vi "Panel.vi"(11 "NumRangeBoolEditorPanel in":refnum<class "NumRangeBoolEditorPanel.lvclass">) -> ()   [LabVIEW 2020, in "VolatusGUIControls.lvlib" / "NumRangeBoolEditorPanel.lvclass"]
uses:
  NumRangeBoolEditorPanel.lvclass
  NumRangeBoolEditorPanel.lvclass/NumRangeBoolEditorPanel.ctl
  lv-oopanel/OOPanel/Panel/Basic UI State.ctl
  lv-oopanel/OOPanel/Panel/Panel.lvclass
  lv-oopanel/OOPanel/OOPanel.lvlib
  VolatusGUIEditorCore/ElementEditorPanel/ElementEditorPanel.lvclass
  lv-autocomplete/AutoComplete/AutoComplete/AutoComplete.lvclass
  VolatusGUIEditorCore/VolatusGUIEditorCore.lvlib
  C:/dev/lv20CE/relink/volatus-gui-controls/VolatusGUIEditorCore/ElementEditorPanel/ElementEditorPanel.lvclass
  C:/dev/lv20CE/relink/lv-oopanel/OOPanel/Panel/Panel.lvclass
  C:/dev/lv20CE/relink/volatus-gui-controls/VolatusGUIControls/NumRangeBoolEditorPanel/NumRangeBoolEditorPanel.lvclass
panel:
  in  "Top":i32
  in  "Left":i32
  in  "Height":u16
  in  "Width":u16
  in  "Label Text Color":u32(colorbox) caption="Color"
  in  "Label Visible":bool caption="Visible"
  in  "Label":string
  in  "Channel":string
  in  "True Color":u32(colorbox)
  in  "False Color":u32(colorbox)
  in  "High":dbl
  in  "Low":dbl
  # "Label"
  # "Out of Range"
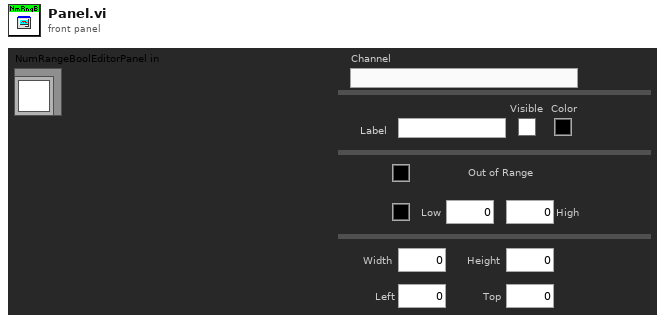
[diagram p1: front panel]
types:
  T1 = typedef "OOPanel.lvlib/Panel.lvclass/Basic UI State.ctl" = enum16{"Init", "Run", "Close"}
  T2 = typedef "VolatusGUIEditorCore.lvlib/ElementEditorPanel.lvclass/Incoming Events.ctl" = cluster{"Update Control":refnum<user-event>}
  T3 = typedef "OOPanel.lvlib/Panel.lvclass/Panel Events.ctl" = cluster{"Visbility":refnum<user-event>, "Close":refnum<user-event>}
  T4 = typedef "VolatusGUIControls.lvlib/NumRangeBoolEditorPanel.lvclass/Props.ctl" = cluster{"JSON":T5, "Label Props":T6, "Position Props":T7, "Boolean Colors Props":T8, "Width":u16, "Height":u16}
  T5 = typedef "VolatusGUIControls.lvlib/NumRangeBoolEditorPanel.lvclass/JSON Props.ctl" = cluster{"Channel":string, "Low":dbl, "High":dbl}
  T6 = typedef "VolatusGUIEditorCore.lvlib/Label Props.ctl" = cluster{"Text":string, "Text Color":u32, "Visible":bool}
  T7 = typedef "VolatusGUIEditorCore.lvlib/Position Props.ctl" = cluster{"Left":i32, "Top":i32}
  T8 = typedef "VolatusGUIEditorCore.lvlib/Boolean Color Props.ctl" = cluster{"False":u32, "True":u32}
  T9 = typedef "OOPanel.lvlib/Visibility State.ctl" = enum16{"Idle", "Closed", "Hidden", "Visible", "Subpanel", "Hidden Subpanel"}
  T10 = cluster{"Label":string, "Label Text Color":u32, "Label Visible":bool}
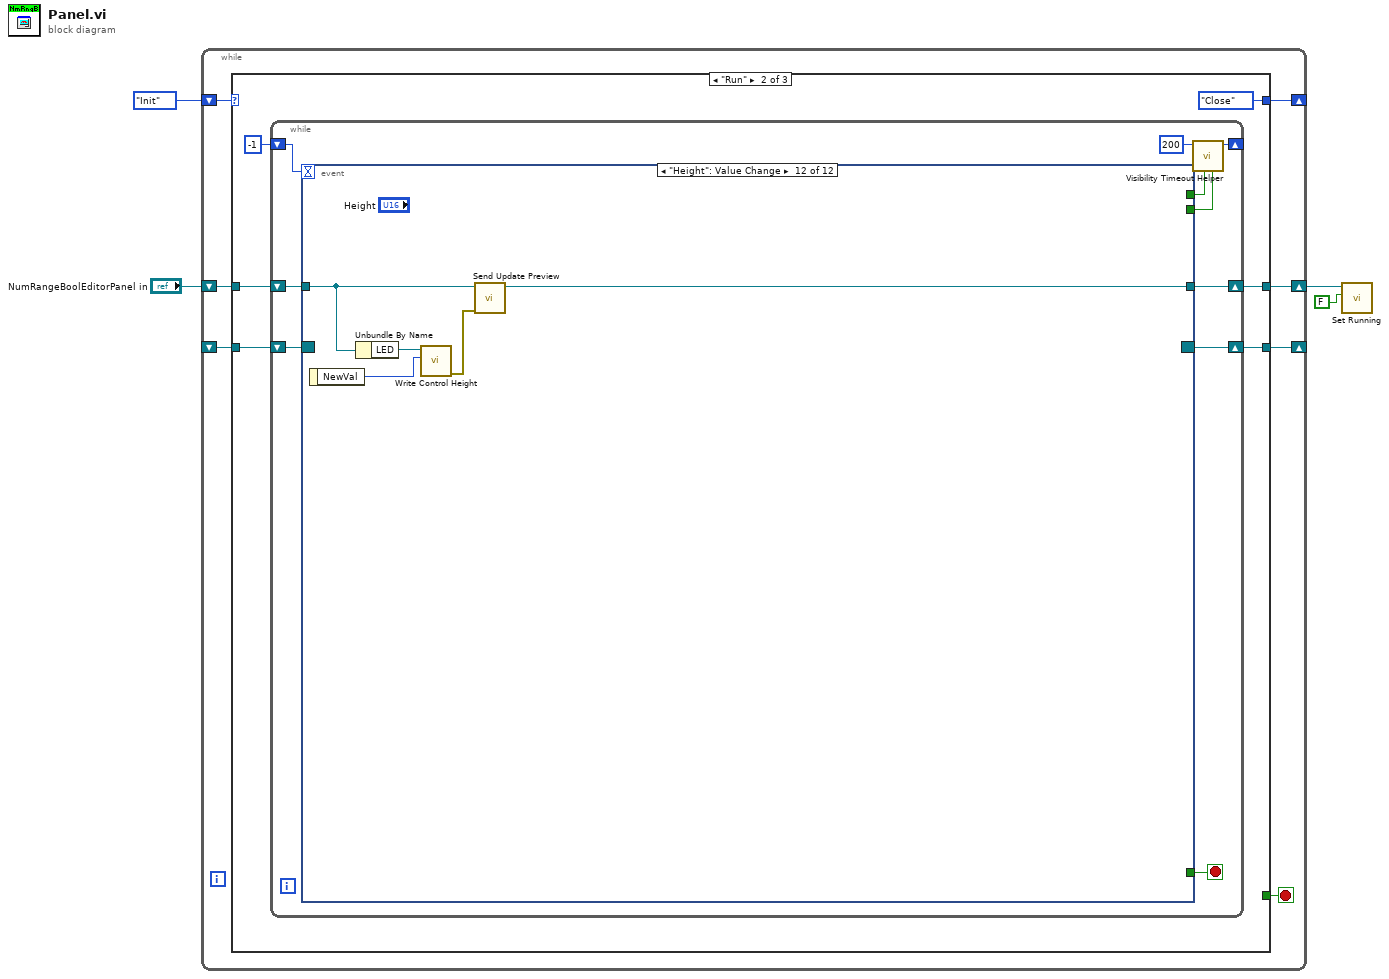
[diagram p0: block diagram]
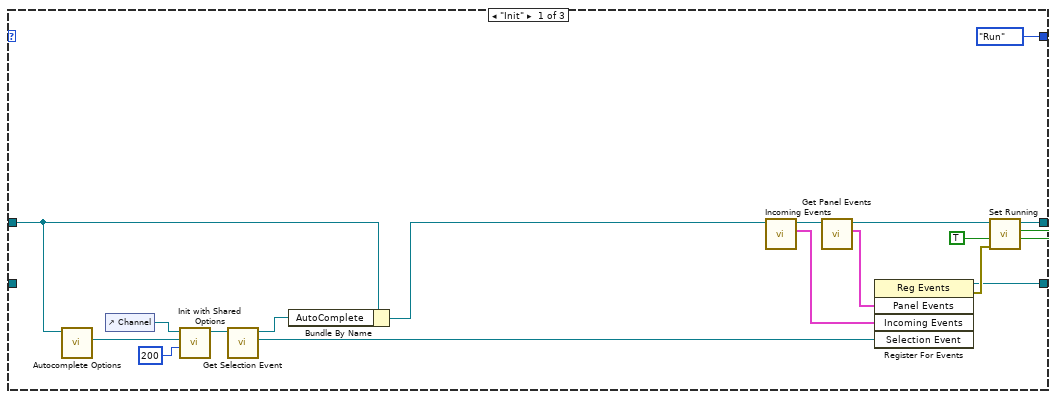
[diagram p2: hidden frame]
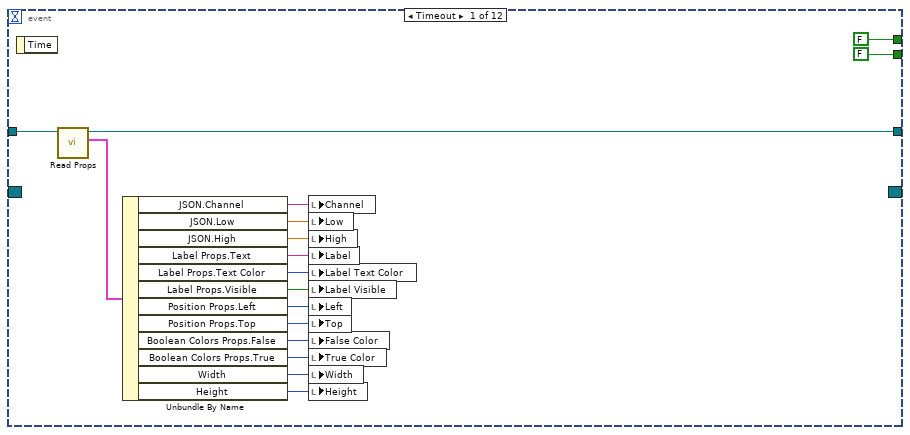
[diagram p3: hidden frame]
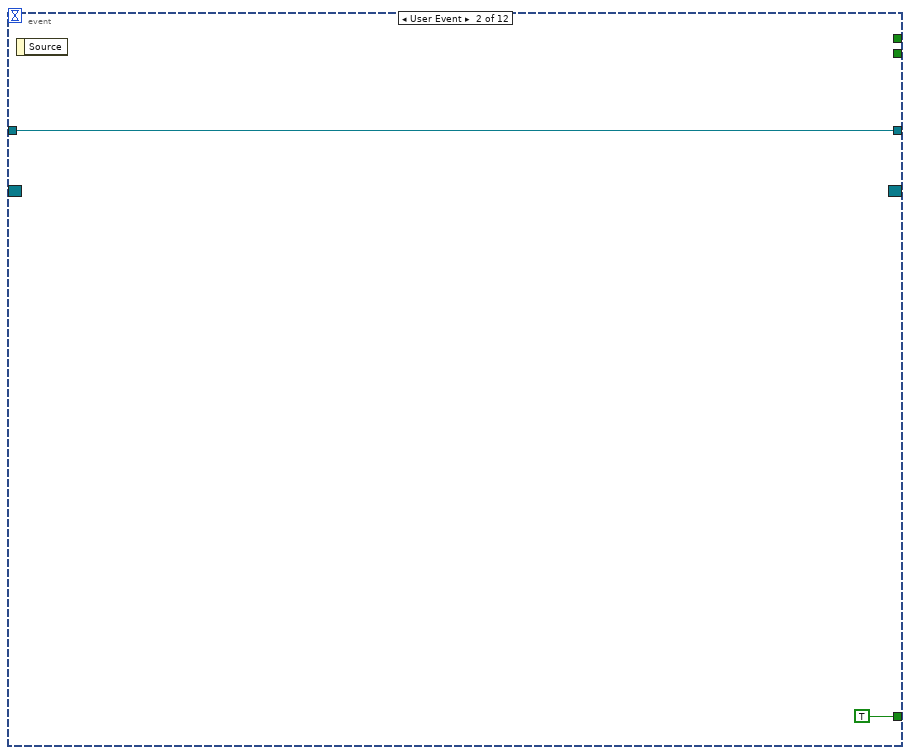
[diagram p4: hidden frame]
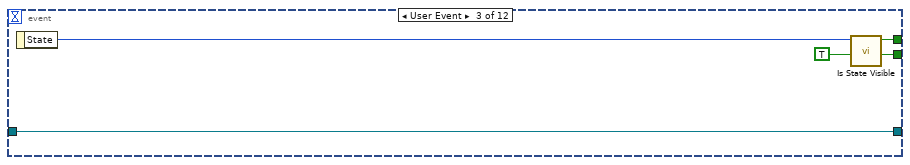
[diagram p5: hidden frame]
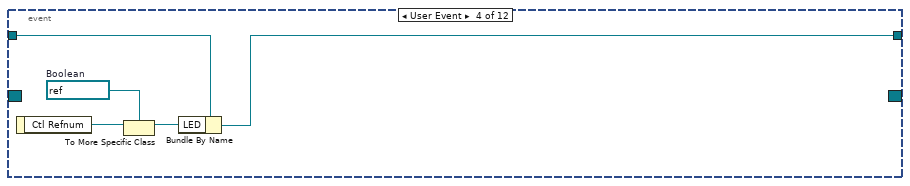
[diagram p6: hidden frame]
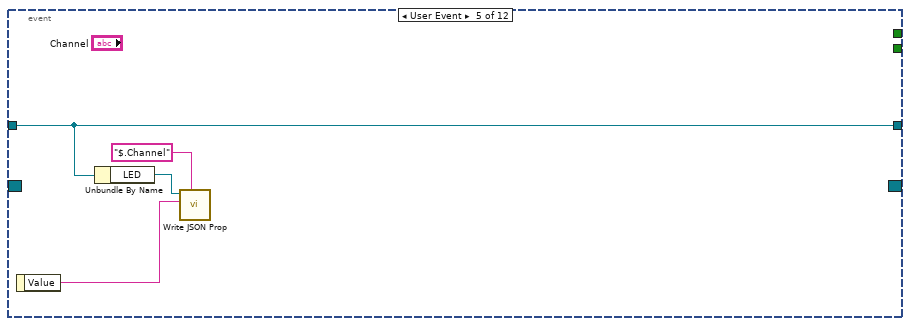
[diagram p7: hidden frame]
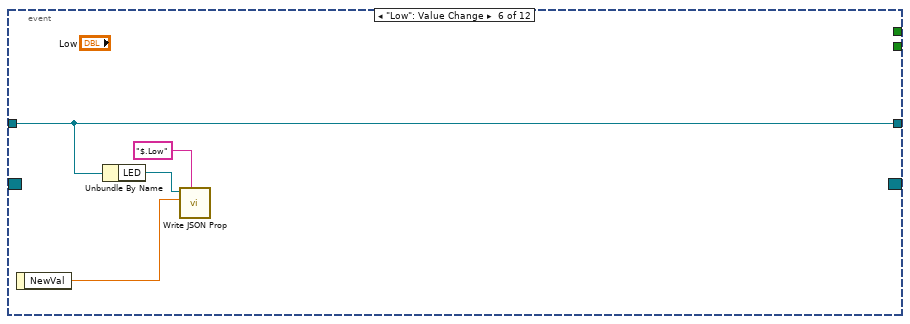
[diagram p8: hidden frame]
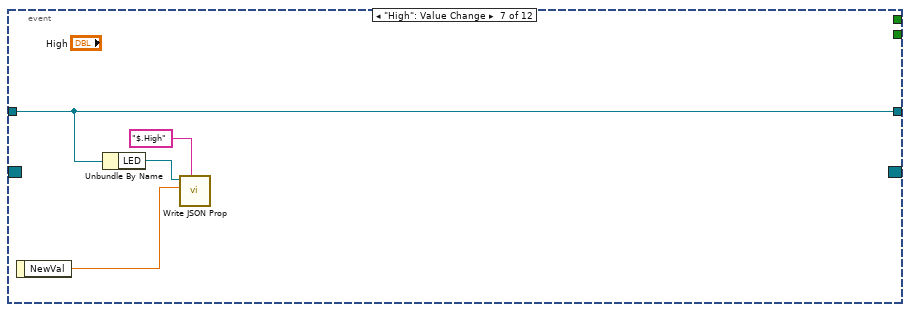
[diagram p9: hidden frame]
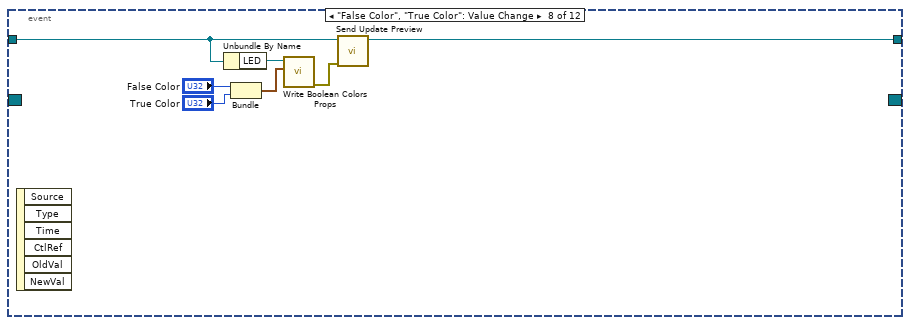
[diagram p10: hidden frame]
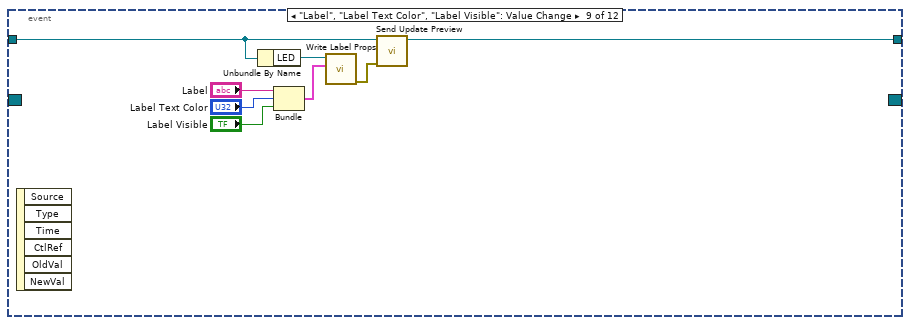
[diagram p11: hidden frame]
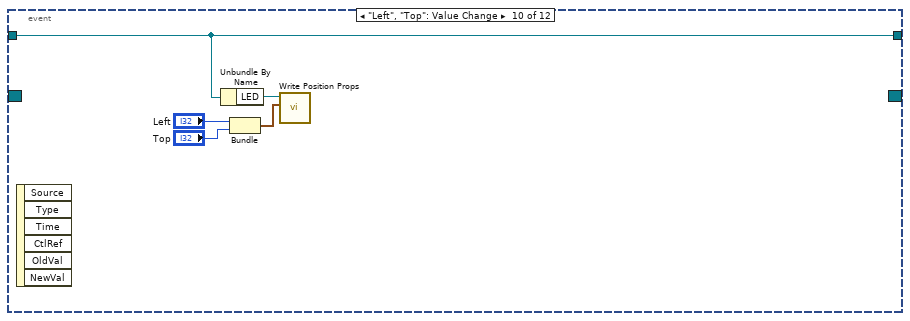
[diagram p12: hidden frame]
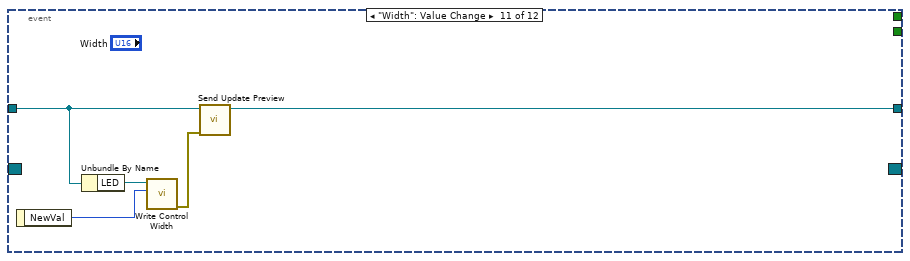
[diagram p13: hidden frame]
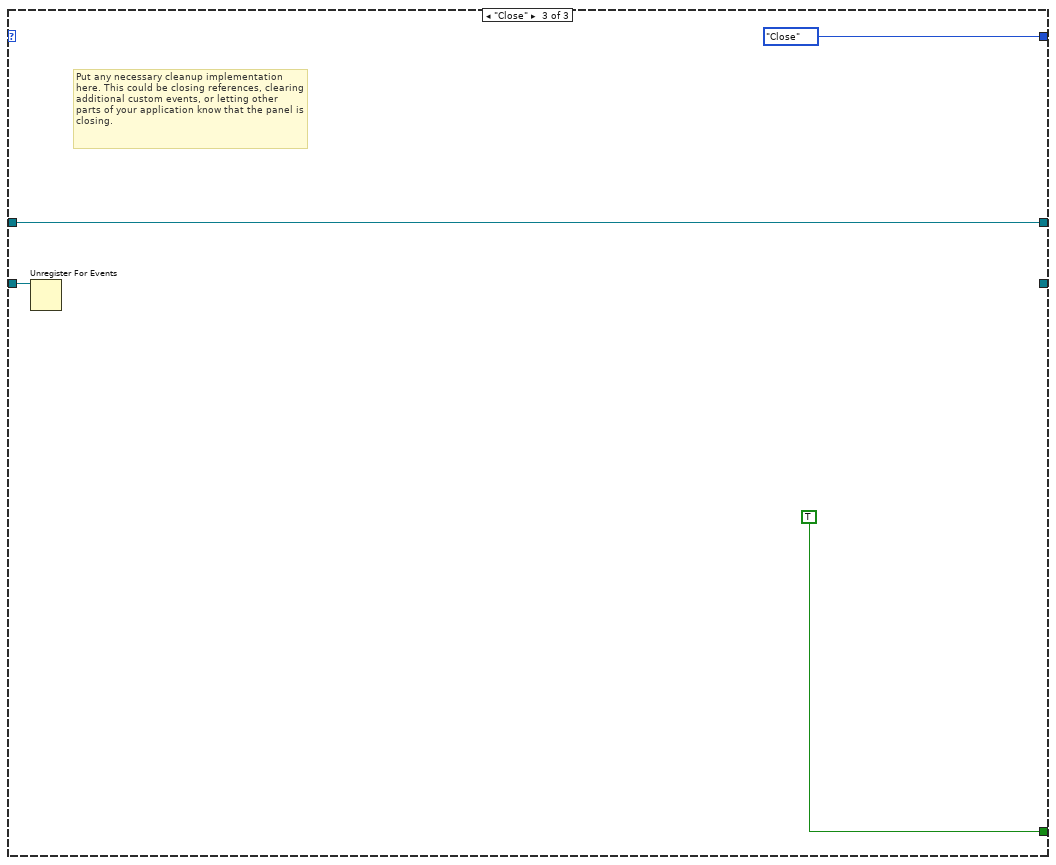
[diagram p14: hidden frame]
diagram:
  n1 = while {
    shift-right: [w10] -> _
    shift-left: _ -> [w11]
    shift-right: [w8] -> _
    shift-left: Basic_UI_State."Init" ("Basic UI State") -> [w9]
    shift-right: [w6] -> w4
    shift-left: "NumRangeBoolEditorPanel in" -> [w5]
    stop <- w7 stop-if-true
    n2 = case shown="\"Run\"" w9 {
      tunnel: w11 -> [_ w34 w116]
      tunnel: [w25 w32 _] -> w10
      tunnel: [Basic_UI_State."Run" ("Basic UI State") Basic_UI_State."Close" ("Basic UI State") Basic_UI_State."Close" ("Basic UI State")] -> w8
      tunnel: [_ _ TRUE] -> w7
      tunnel: [w24 w29 w115] -> w6
      tunnel: w5 -> [w17 w30 w115]
      frame "Init" {
        n3 = call "Autocomplete Options.vi"("ElementEditorPanel in"=w17) -> ("Autocomplete Options"=w19:refnum<class "Shared Options.lvclass">)  [unwired: 10 in]
        n4 = control-ref of="Channel"() -> (w16:refnum<vi>)
        n5 = call "Init with Shared Options.vi"("Height (200)"=i16 200, "Shared Options"=w19, "Str Refnum"=w16) -> ("AutoComplete out"=w15:refnum<class "AutoComplete.lvclass">)  [unwired: 7 in, 1 out]
        n6 = call "Get Selection Event.vi"("AutoComplete in"=w15) -> ("Selection Event"=w14:refnum<user-event>, "AutoComplete"=w12:refnum<class "AutoComplete.lvclass">)  [unwired: 9 in]
        n7 = Bundle By Name(cluster=w17, "AutoComplete"=w12) -> (w13:refnum<class "NumRangeBoolEditorPanel.lvclass">)
        n8 = call "Incoming Events.vi"("ElementEditorPanel in"=w13) -> ("Incoming Events"=w20:T2, "ElementEditorPanel out"=w21:refnum<class "NumRangeBoolEditorPanel.lvclass">)  [unwired: 9 in]
        n9 = call "Get Panel Events.vi"("Panel in"=w21) -> ("Panel Events"=w22:T3, "Panel out"=w23:refnum<class "NumRangeBoolEditorPanel.lvclass">)  [unwired: 8 in, 1 out]
        n10 = register-events(w22, w20, w14) -> (reference out=w25:refnum<event-registration>, error out=w27:errorcluster)  [unwired: 2 in]
        n11 = call "Set Running.vi"("error in (no error)"=w27, "Running"=TRUE, "Panel in"=w23) -> ("Panel out"=w24:refnum<class "NumRangeBoolEditorPanel.lvclass">)  [unwired: 7 in, 1 out]
      }
      frame "Run" {
        n12 = while {
          shift-right: [w40] -> w32
          shift-left: w34 -> [w41]
          shift-right: [w43] -> _
          shift-left: -1 ("Timeout") -> [w42]
          shift-right: [w35] -> w29
          shift-left: w30 -> [w36]
          stop <- w37 stop-if-true
          n13 = event shown="[11] \"Height\": Value Change" {
            selector: w41 -> [_ _ _ _ _ _ _ _ _ _ _ _]
            dyn-events: [_ _ _ _ _ _ _ _ _ _ _ _] -> w40
            timeout: w42 -> [_ _ _ _ _ _ _ _ _ _ _ _]
            tunnel: [FALSE _ w66 _ _ _ _ _ _ _ _ _] -> w39
            tunnel: [FALSE _ TRUE _ _ _ _ _ _ _ _ _] -> w38
            tunnel: [_ TRUE _ _ _ _ _ _ _ _ _ _] -> w37
            tunnel: w36 -> [w58 w62 w64 w72 w74 w78 w82 w88 w96 w101 w108 w113]
            tunnel: [w59 w62 w64 w69 w74 w78 w82 w86 w93 w101 w106 w111] -> w35
            event Timeout {
              n14 = event-data() -> ()  [unwired: 1 in, 1 out]
              n15 = call "Read Props.vi"("NumRangeBoolEditorPanel in"=w58) -> ("Props"=w57:T4, "NumRangeBoolEditorPanel out"=w59:refnum<class "NumRangeBoolEditorPanel.lvclass">)  [unwired: 8 in, 1 out]
              n16 = Unbundle By Name(w57) -> ("JSON.Channel"=w56:string, "JSON.Low"=w54:dbl, "JSON.High"=w53:dbl, "Label Props.Text"=w52:string, "Label Props.Text Color"=w51:u32, "Label Props.Visible"=w50:bool, "Position Props.Left"=w49:i32, "Position Props.Top"=w48:i32, "Boolean Colors Props.False"=w47:u32, "Boolean Colors Props.True"=w46:u32, "Width"=w45:u16, "Height"=w55:u16)
              n17 = local write "Channel"(w56) -> ()
              n18 = local write "Low"(w54) -> ()
              n19 = local write "High"(w53) -> ()
              n20 = local write "Label"(w52) -> ()
              n21 = local write "Label Text Color"(w51) -> ()
              n22 = local write "Label Visible"(w50) -> ()
              n23 = local write "Left"(w49) -> ()
              n24 = local write "Top"(w48) -> ()
              n25 = local write "False Color"(w47) -> ()
              n26 = local write "True Color"(w46) -> ()
              n27 = local write "Width"(w45) -> ()
              n28 = local write "Height"(w55) -> ()
            }
            event User Event {
              n29 = event-data() -> ()  [unwired: 1 in, 1 out]
            }
            event User Event {
              n30 = event-data() -> ("State"=w67:T9)  [unwired: 1 in]
              n31 = call "Is State Visible.vi"("Visibility"=w67) -> ("Visible"=w66:bool)  [unwired: 10 in]
            }
            event User Event {
              w70 = refnum<vi> refnum  # Boolean
              n32 = event-data() -> ("Ctl Refnum"=w71:refnum<vi>)  [unwired: 1 in]
              n33 = To More Specific Class(target class=w70, reference=w71) -> (specific class reference=w68:refnum<vi>)  [unwired: 1 in, 1 out]
              n34 = Bundle By Name(cluster=w72, "LED"=w68) -> (w69:refnum<class "NumRangeBoolEditorPanel.lvclass">)
            }
            event User Event {
              n35 = event-data() -> ("Value"=w73:string)  [unwired: 1 in]
              n36 = Unbundle By Name(w74) -> ("LED"=w76:refnum<vi>)
              n37 = call "Write JSON Prop.vi"("JSON Path"="$.Channel" ("$Path or Item Name"), "Value"=w73, "Ctl Refnum in"=w76) -> ()  [unwired: 7 in, 2 out]
            }
            event "Low": Value Change {
              n38 = event-data() -> ("NewVal"=w77:dbl)  [unwired: 1 in]
              n39 = Unbundle By Name(w78) -> ("LED"=w80:refnum<vi>)
              n40 = call "Write JSON Prop.vi"("JSON Path"="$.Low" ("$Path or Item Name"), "Value"=w77, "Ctl Refnum in"=w80) -> ()  [unwired: 7 in, 2 out]
            }
            event "High": Value Change {
              n41 = event-data() -> ("NewVal"=w81:dbl)  [unwired: 1 in]
              n42 = Unbundle By Name(w82) -> ("LED"=w84:refnum<vi>)
              n43 = call "Write JSON Prop.vi"("JSON Path"="$.High" ("$Path or Item Name"), "Value"=w81, "Ctl Refnum in"=w84) -> ()  [unwired: 7 in, 2 out]
            }
            event "False Color", "True Color": Value Change {
              n44 = event-data() -> ()  [unwired: 1 in, 6 out]
              n45 = Unbundle By Name(w88) -> ("LED"=w87:refnum<vi>)
              n46 = Bundle("False Color"="False Color", "True Color"="True Color") -> (w89:cluster{"False Color":u32, "True Color":u32})  [unwired: 1 in]
              n47 = call "Write Boolean Colors Props.vi"("Boolean Colors Props"=w89, "Control in"=w87) -> ("error out"=w85:errorcluster)  [unwired: 8 in, 1 out]
              n48 = call "Send Update Preview.vi"("error in (no error)"=w85, "ElementEditorPanel in"=w88) -> ("ElementEditorPanel out"=w86:refnum<class "NumRangeBoolEditorPanel.lvclass">)  [unwired: 8 in, 1 out]
            }
            event "Label", "Label Text Color", "Label Visible": Value Change {
              n49 = event-data() -> ()  [unwired: 1 in, 6 out]
              n50 = Unbundle By Name(w96) -> ("LED"=w95:refnum<vi>)
              n51 = Bundle("Label"="Label", "Label Text Color"="Label Text Color", "Label Visible"="Label Visible") -> (w94:T10)  [unwired: 1 in]
              n52 = call "Write Label Props.vi"("Label Props"=w94, "Ctl Refnum in"=w95) -> ("error out"=w92:errorcluster)  [unwired: 8 in, 1 out]
              n53 = call "Send Update Preview.vi"("error in (no error)"=w92, "ElementEditorPanel in"=w96) -> ("ElementEditorPanel out"=w93:refnum<class "NumRangeBoolEditorPanel.lvclass">)  [unwired: 8 in, 1 out]
            }
            event "Left", "Top": Value Change {
              n54 = event-data() -> ()  [unwired: 1 in, 6 out]
              n55 = Unbundle By Name(w101) -> ("LED"=w100:refnum<vi>)
              n56 = Bundle("Left"="Left", "Top"="Top") -> (w102:cluster{"Left":i32, "Top":i32})  [unwired: 1 in]
              n57 = call "Write Position Props.vi"("Position Props"=w102, "Ctl Refnum in"=w100) -> ()  [unwired: 8 in, 2 out]
            }
            event "Width": Value Change {
              n58 = event-data() -> ("NewVal"=w109:u16)  [unwired: 1 in]
              n59 = Unbundle By Name(w108) -> ("LED"=w107:refnum<vi>)
              n60 = call "Write Control Width.vi"("Width"=w109, "Control in"=w107) -> ("error out"=w105:errorcluster)  [unwired: 8 in, 1 out]
              n61 = call "Send Update Preview.vi"("error in (no error)"=w105, "ElementEditorPanel in"=w108) -> ("ElementEditorPanel out"=w106:refnum<class "NumRangeBoolEditorPanel.lvclass">)  [unwired: 8 in, 1 out]
            }
            event "Height": Value Change {
              n62 = event-data() -> ("NewVal"=w114:u16)  [unwired: 1 in]
              n63 = Unbundle By Name(w113) -> ("LED"=w112:refnum<vi>)
              n64 = call "Write Control Height.vi"("Height"=w114, "Control in"=w112) -> ("error out"=w110:errorcluster)  [unwired: 8 in, 1 out]
              n65 = call "Send Update Preview.vi"("error in (no error)"=w110, "ElementEditorPanel in"=w113) -> ("ElementEditorPanel out"=w111:refnum<class "NumRangeBoolEditorPanel.lvclass">)  [unwired: 8 in, 1 out]
            }
          }
          n66 = call "Visibility Timeout Helper.vi"("Update?"=w38, "Use Timeout?"=w39, "Visible Timeout mS"=200) -> ("Timeout"=w43:i32)  [unwired: 8 in]
        }
      }
      frame "Close" {
        # "Put any necessary cleanup implementation here. This could be closing references, clearing additional custom events, or letting other parts of your application know that the panel is closing."
        n67 = Unregister For Events(event registration refnum=w116) -> ()  [unwired: 1 in, 1 out]
      }
    }
  }
  n68 = call "Set Running.vi"("Running"=FALSE, "Panel in"=w4) -> ()  [unwired: 8 in, 2 out]
